vi "Host - Get Slave IOVs.vi"(8 "error in (no error)":errorcluster, 11 "ECAT Master in":refnum<k21>) -> (0 "error IO":errorcluster, 2 "All Slaves":refnum<k21>[](array[refnum]), 3 "ECAT Master out":refnum<k21>)   [LabVIEW 2019, in "SEECD System Explorer.lvlib"]
uses:
  SEECD System Explorer.lvlib
  <resource>/objmgr/IndComECAT.rc
  Shared/SEECD Shared.lvlib
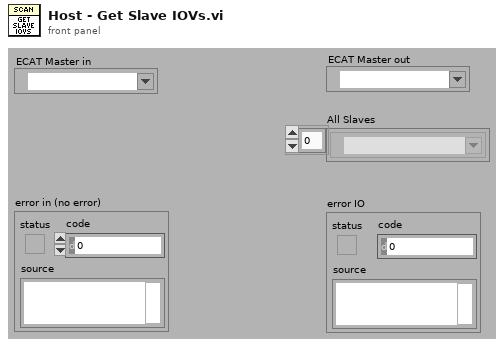
[diagram p1: front panel]
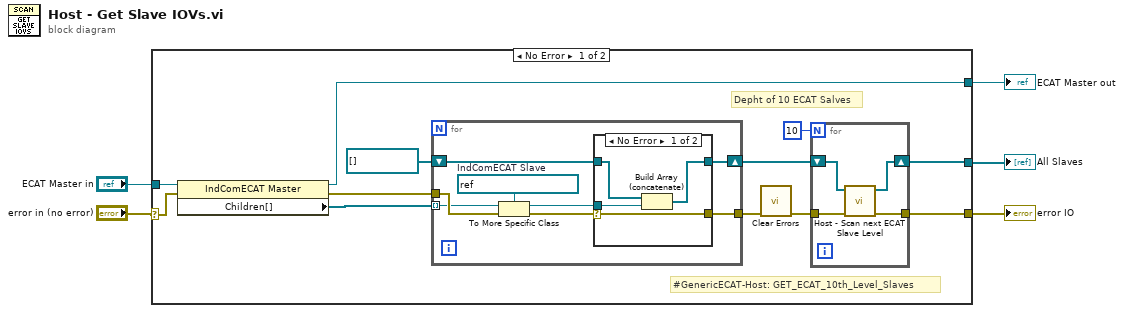
[diagram p0: block diagram]
diagram:
  n1 = case shown="No Error" "error in (no error)" {
    selector: "error in (no error)" -> [w15 w37]
    tunnel: [w6 w37] -> w5
    tunnel: [w7 _] -> w4
    tunnel: "ECAT Master in" -> [w17 w36]
    tunnel: [w16 w36] -> w2
    frame No Error {
      # "Depht of 10 ECAT Salves"
      # "#GenericECAT-Host: GET_ECAT_10th_Level_Slaves"
      n2 = property class="IndComECAT Master"(reference=w17, error in=w15) -> (reference out=w16:refnum<k21>, error out=w12:errorcluster, "Children[]"=w13:refnum<k21>[])
      n3 = for {
        tunnel: w13 -> [w28] mode=indexing
        tunnel: w12 -> [w29]
        shift-right: [w26] -> w9
        shift-left: refnum<k21>[] [] -> [w25]
        tunnel: [w24] -> w10
        w27 = refnum<k21> refnum  # IndComECAT Slave
        n4 = To More Specific Class(target class=w27, reference=w28, error in=w29) -> (specific class reference=w22:refnum<k21>, error out=w23:errorcluster)
        n5 = case shown="No Error" w23 {
          selector: w23 -> [w30 w34]
          tunnel: w22 -> [w33 _]
          tunnel: [w32 w35] -> w26
          tunnel: w25 -> [w31 w35]
          tunnel: [w30 w34] -> w24
          frame No Error {
            n6 = Build Array (concatenate)(w31, w33) -> (w32:refnum<k21>[])
          }
          frame Error {
          }
        }
      }
      n7 = call <vilib>:"Clear Errors.vi"("error in (no error)"=w10) -> ("error out"=w11:errorcluster)  [unwired: 5 in, 1 out]
      n8 = for {
        N: 10 -> [_]
        tunnel: w11 -> [w21]
        tunnel: [w18] -> w6
        shift-right: [w19] -> w7
        shift-left: w9 -> [w20]
        n9 = call "Host - Scan next ECAT Slave Level.vi"("Fehler (Eingang, kein Fehler)"=w21, "Array (Eingang)"=w20) -> ("Fehler (Ausgang)"=w18:errorcluster, "Array (Ausgang)"=w19:refnum<k21>[])  [unwired: 8 in]
      }
    }
    frame Error {
    }
  }
  "All Slaves" <- w4
  "error IO" <- w5
  "ECAT Master out" <- w2
